vi "PR_Update_Assemble_result  .vi"(8 "error in (no error)":errorcluster, 9 "screw_result":string, 10 "barcode":string="123465798", 11 "DBlink":string="Driver={ODBC Driver 17 for SQL Server};Server=localhost\\SQLEXPRESS;Database=ZDX201;UID=labview;PWD=Dsa@54137926") -> (0 "error out":errorcluster)   [LabVIEW 2019]
uses:
  <vilib>/addons/database/Connection.llb/DB Tools Open Connec (String).vi
  <vilib>/addons/database/NI_Database_API.lvlib
panel:
  out "concatenated string":string="WHERE [barcode]='984132195' and [pos]='B'"
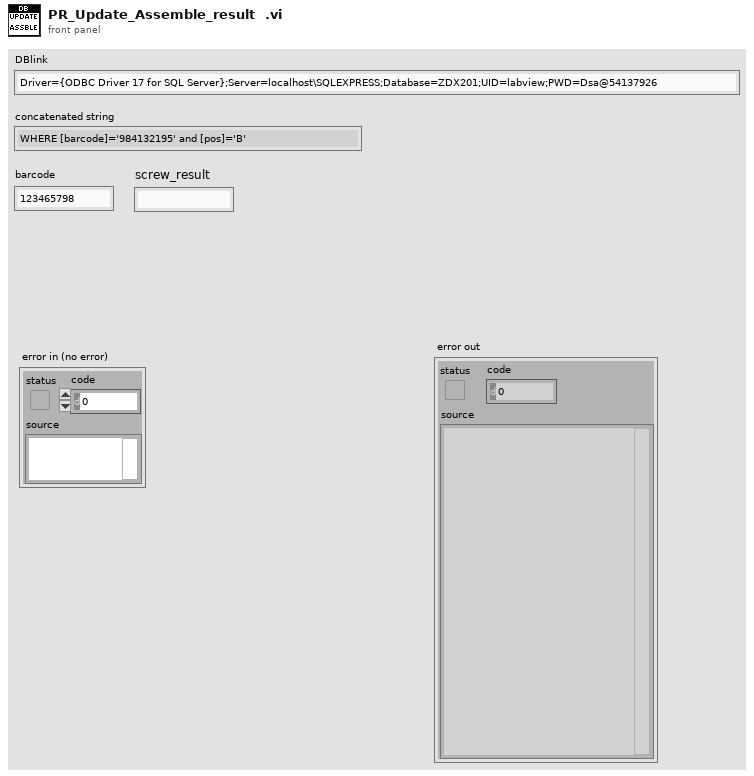
[diagram p1: front panel]
types:
  T1 = cluster{"screw_result":string, "update_time":timestamp}
  T2 = typedef "NI_Database_API.lvlib/Conn ObjectReference.ctl" = refnum<k1>
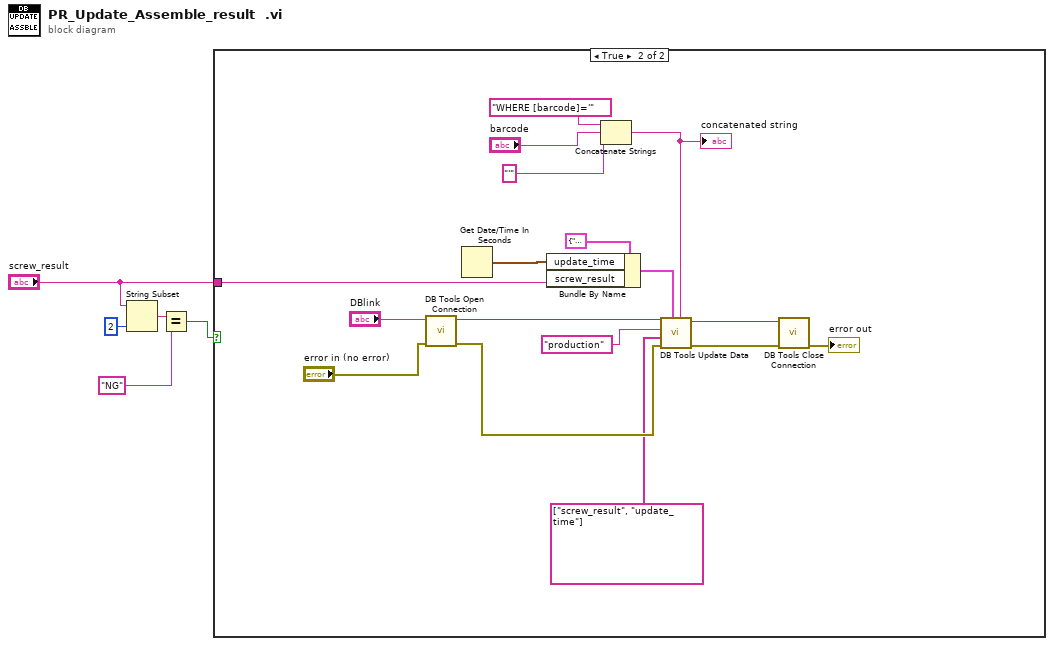
[diagram p0: block diagram]
diagram:
  n1 = String Subset(string="screw_result", length (rest)=2 ("length (rest)")) -> (substring=w3:string)  [unwired: 1 in]
  n2 = Equal?(x=w3, y="NG") -> (x = y?=w1:bool)
  n3 = case shown="True" w1 {
    tunnel: "screw_result" -> [_ w6]
    frame False {
    }
    frame True {
      n4 = call-poly <vilib>:"DB Tools Open Connection.vi"("error in (no error)"="error in (no error)", "connection information"="DBlink") -> ("error out"=w20:errorcluster, "connection reference"=w18:T2)  [unwired: 6 in]
      n5 = Get Date/Time In Seconds() -> (seconds since 1Jan1904=w8:timestamp)
      n6 = Bundle By Name(cluster=T1 {"screw_result"="", "update_time"=timestamp(0 s since 1904-01-01)}, "update_time"=w8, "screw_result"=w6) -> (w7:T1)
      n7 = Concatenate Strings("WHERE [barcode]='", "barcode", "'" ("string")) -> (w12:string)
      "concatenated string" <- w12
      n8 = call <vilib>:"DB Tools Update Data.vi"("condition"=w12, "data"=w7, "error in (no error)"=w20, "columns"=string[] ["screw_result", "update_time"], "table"="production", "connection reference"=w18) -> ("error out"=w21:errorcluster, "connection reference out"=w19:T2)  [unwired: 4 in]
      n9 = call <vilib>:"DB Tools Close Connection.vi"("error in (no error)"=w21, "connection reference"=w19) -> ("error out"=→"error out":errorcluster)  [unwired: 5 in]
    }
  }
